vi "While condition.vi"   [LabVIEW 2020, in "Exaprom PDF.lvlib"]
uses:
  <userlib>/labview-PDF-writer-master/Exaprom PDF.lvlib
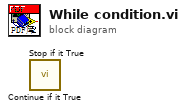
[diagram p0: block diagram]
diagram:
  n1 = call <userlib>:"Continue if it True.vi"() -> ()  [unwired: 7 in, 2 out]
  n2 = call <userlib>:"Stop if it True.vi"() -> ()  [unwired: 7 in, 2 out]
